vi "calc energy stats.vi"(0 "integration cluster":T2, 5 "z0":dbl=0.0492, 7 "m":dbl=0.5526, 9 "g":dbl=9.802, 11 "lifetime":dbl=1000.0) -> (4 "output cluster":T1 {"Uavg" format="%_3p"; "Uloss" format="%_3p"; "Uloss_avg" format="%_3p"; "Upulse" format="%_3p"; "Upulse_avg" format="%_3p"; "DeltaU" format="%_3p"; "DeltaU_avg" format="%_3g"}, 6 "T":dbl, 8 "L":dbl, 10 "Uinst":dbl, 14 "Ufinal":dbl, 15 "Uinit":dbl)   [LabVIEW 2017]
uses:
  popup panels/control panel globals.vi
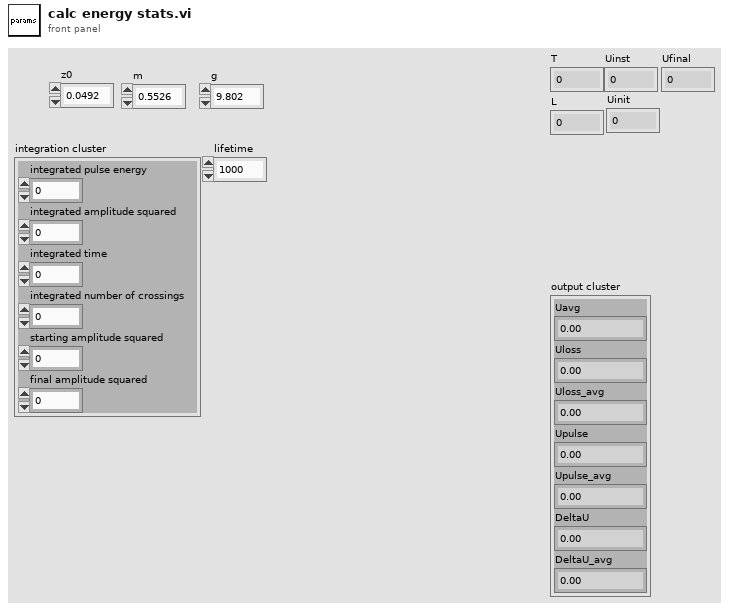
[diagram p1: front panel]
types:
  T1 = cluster{"Uavg":dbl, "Uloss":dbl, "Uloss_avg":dbl, "Upulse":dbl, "Upulse_avg":dbl, "DeltaU":dbl, "DeltaU_avg":dbl}
  T2 = cluster{"integrated pulse energy":dbl, "integrated amplitude squared":dbl, "integrated time":dbl, "integrated number of crossings":dbl, "starting amplitude squared":dbl, "final amplitude squared":dbl}
  T3 = typedef "magnetic field fit.ctl" = cluster{"a":dbl, "b":dbl, "theta":dbl, "scaling":dbl, "tilt_x":dbl, "tilt_y":dbl, "bx_offset":dbl, "by_offset":dbl, "bz_offset":dbl, "x_offset":dbl, "y_offset":dbl}
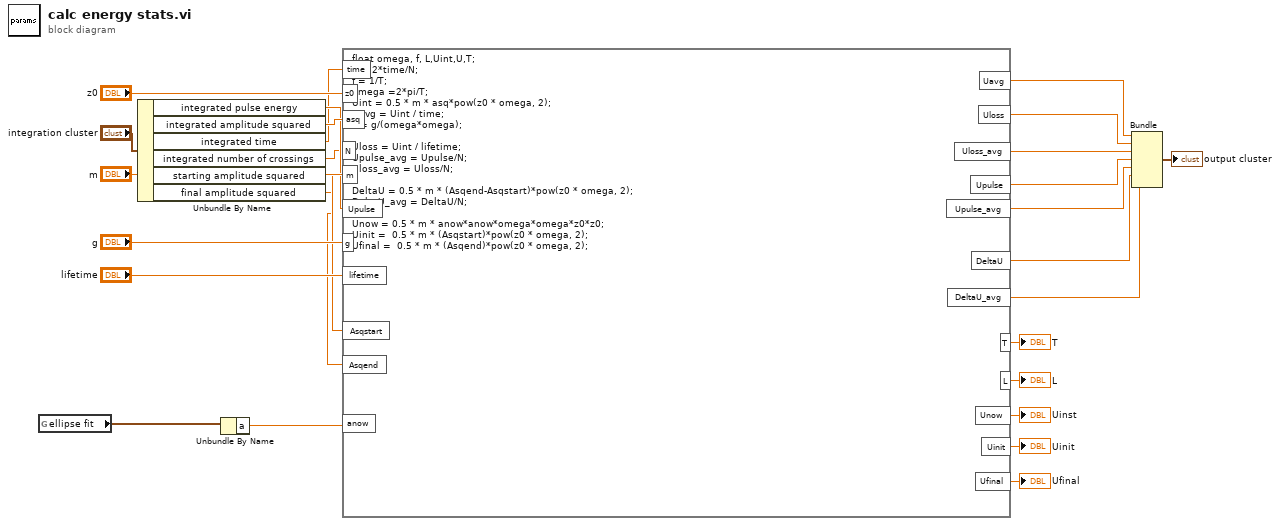
[diagram p0: block diagram]
diagram:
  n1 = global read "control panel globals.vi" "ellipse fit"() -> (w5:T3)
  n2 = Unbundle By Name("integration cluster") -> ("integrated pulse energy"=w16:dbl, "integrated amplitude squared"=w17:dbl, "integrated time"=w15:dbl, "integrated number of crossings"=w14:dbl, "starting amplitude squared"=w12:dbl, "final amplitude squared"=w11:dbl)
  n3 = Unbundle By Name(w5) -> ("a"=w4:dbl)
  n4 = formula code="float omega, f, L,Uint,U,T;\nT = 2*time/N;\nf = 1/T;\nomega =2*pi/T;\nUint = 0.5 * m * asq*pow(z0 * omega, 2);\nUavg = Uint / time;\nL = g/(omega*omega);\n\nUloss = Uint / lifetime;\nUpulse_avg = Upulse/N;\nUloss_avg = Uloss/N;\n\nDeltaU = 0.5 * m * (Asqend-Asqstart)*pow(z0 * omega, 2);\nDeltaU_avg = DeltaU/N;\n\nUnow = 0.5 * m * anow*anow*omega*omega*z0*z0;\nUinit =  0.5 * m * (Asqstart)*pow(z0 * omega, 2);\nUfinal =  0.5 * m * (Asqend)*pow(z0 * omega, 2);"("time"=w15, "z0"="z0", "asq"=w17, "N"=w14, "m"="m", "Upulse"=w16, "g"="g", "lifetime"="lifetime", "Asqstart"=w12, "Asqend"=w11, "anow"=w4) -> ("Uavg"=w24:dbl, "Uloss"=w23:dbl, "Uloss_avg"=w22:dbl, "Upulse"=w21:dbl, "Upulse_avg"=w20:dbl, "DeltaU"=w10:dbl, "DeltaU_avg"=w9:dbl, "T"=→"T":dbl, "L"=→"L":dbl, "Unow"=→"Uinst":dbl, "Uinit"=→"Uinit":dbl, "Ufinal"=→"Ufinal":dbl)
  n5 = Bundle("Uavg"=w24, "Uloss"=w23, "Uloss_avg"=w22, "Upulse"=w21, "Upulse_avg"=w20, "DeltaU"=w10, "DeltaU_avg"=w9) -> (→"output cluster":T1)  [unwired: 1 in]
